vi "scan.vi"() -> (1 "载具码":string)   [LabVIEW 2014]
panel:
  in  "退出":bool
  in  "扫码控制键":bool
  in  "识别载具信息":string
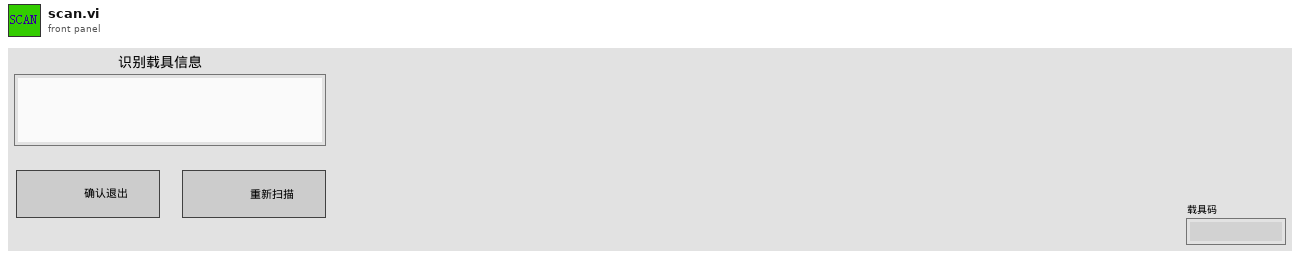
[diagram p1: front panel]
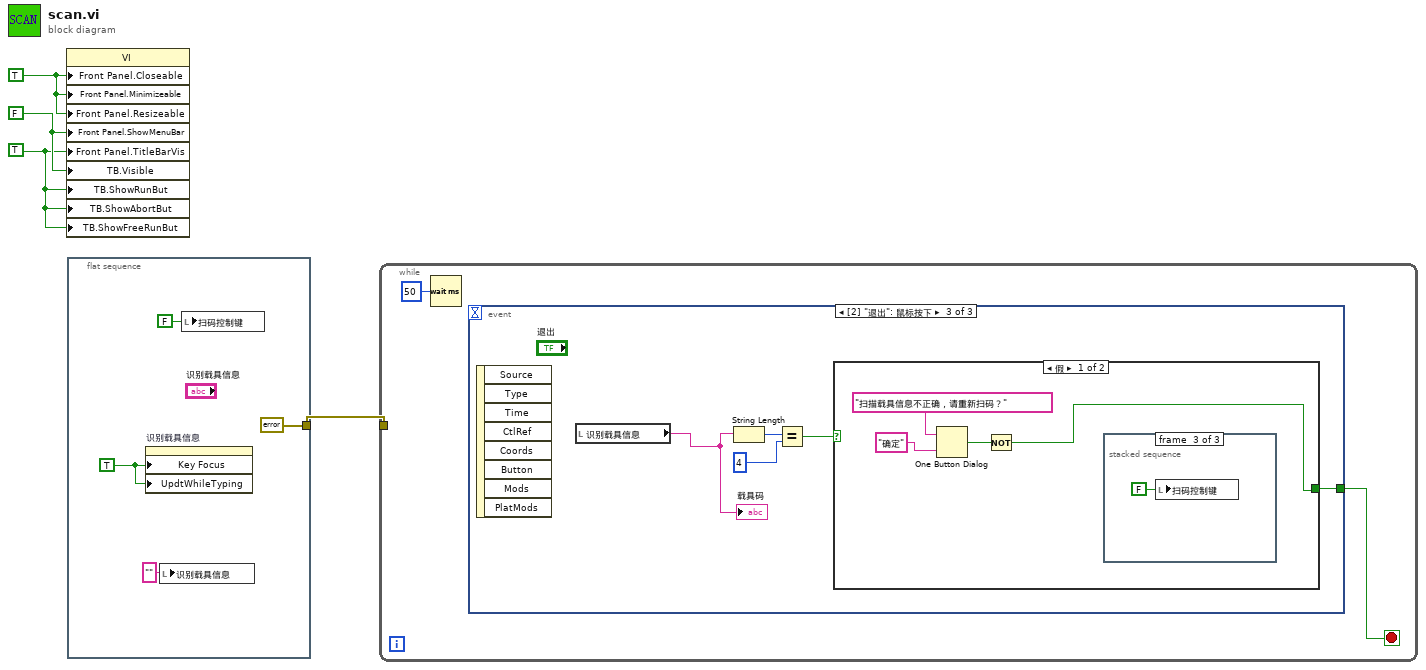
[diagram p0: block diagram]
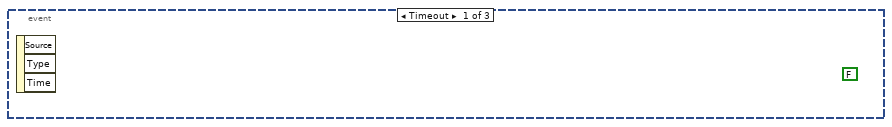
[diagram p2: hidden frame]
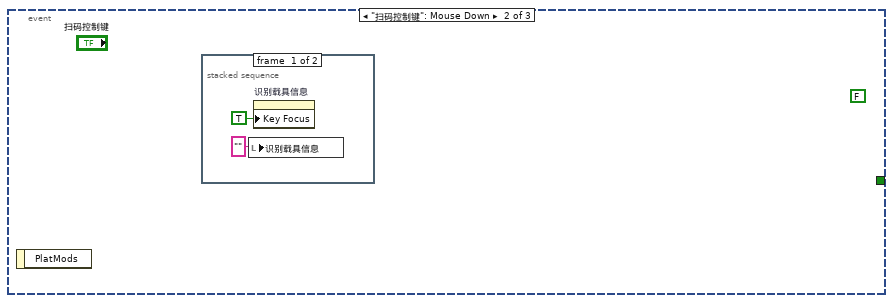
[diagram p3: hidden frame]
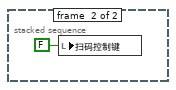
[diagram p4: hidden frame]
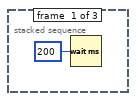
[diagram p5: hidden frame]
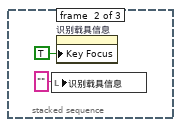
[diagram p6: hidden frame]
diagram:
  w2 = TRUE ("前面板窗口:可关闭")
  w1 = TRUE ("前面板窗口:可关闭")
  w3 = FALSE ("Front Panel Window:Closeable")
  n1 = property class="VI"("Front Panel.Closeable"=w1, "Front Panel.Minimizeable"=w1, "Front Panel.Resizeable"=w1, "Front Panel.ShowMenuBar"=w3, "Front Panel.TitleBarVis"=w2, "TB.Visible"=w3, "TB.ShowRunBut"=w2, "TB.ShowAbortBut"=w2, "TB.ShowFreeRunBut"=w2) -> ()  [unwired: 2 in, 2 out]
  n2 = flat-sequence {
    tunnel: [errorcluster {"status"=FALSE, "code"=0, "source"=""} ("错误常量")] -> w4
    frame #0 {
      w5 = TRUE ("键选中")
      n3 = property on="识别载具信息" class="Str"("Key Focus"=w5, "UpdtWhileTyping"=w5) -> ()  [unwired: 2 in, 2 out]
      n4 = local write "识别载具信息"("" ("扫码信息")) -> ()
      n5 = local write "扫码控制键"(FALSE ("扫码控制键")) -> ()
    }
  }
  n6 = while {
    tunnel: w4 -> [_]
    stop <- w9 stop-if-true
    n7 = Wait (ms)(milliseconds to wait=u32 50 ("等待时间（毫秒）")) -> ()  [unwired: 1 out]
    n8 = event shown="[2] \"退出\": 鼠标按下" {
      selector: _ -> [_ _ _]
      dyn-events: _ -> [_ _ _]
      timeout: _ -> [_ _ _]
      tunnel: [_ _ w18] -> w9
      event Timeout {
        (unwired) FALSE
        n9 = event-data() -> ()  [unwired: 1 in, 3 out]
      }
      event "扫码控制键": Mouse Down {
        (unwired) FALSE
        n10 = event-data() -> ()  [unwired: 1 in, 1 out]
        n11 = stacked-sequence {
          frame #0 {
            n12 = local write "识别载具信息"("" ("扫码信息")) -> ()
            n13 = property on="识别载具信息" class="Str"("Key Focus"=TRUE ("键选中")) -> ()  [unwired: 2 in, 2 out]
          }
          frame #1 {
            n14 = local write "扫码控制键"(FALSE ("扫码控制键")) -> ()
          }
        }
      }
      event "退出": Mouse Down {
        n15 = event-data() -> ()  [unwired: 1 in, 8 out]
        n16 = local read "识别载具信息"() -> (w14:string)
        "载具码" <- w14
        n17 = String Length(string=w14) -> (length=w16:i32)
        n18 = Equal?(x=w16, y=4) -> (x = y?=w17:bool)
        n19 = case shown="假" w17 {
          selector: w17 -> [_ w27]
          tunnel: [w22 w27] -> w18
          frame False {
            n20 = One Button Dialog(message="扫描载具信息不正确，请重新扫码？" ("消息"), button name ("OK")="确定" ("T按钮名称（“确定”）")) -> (true=w19:bool)
            n21 = Not(x=w19) -> (.not. x?=w22:bool)
            n22 = stacked-sequence {
              frame #0 {
                n23 = Wait (ms)(milliseconds to wait=u32 200 ("等待时间（毫秒）")) -> ()  [unwired: 1 out]
              }
              frame #1 {
                n24 = local write "识别载具信息"("" ("扫码信息")) -> ()
                n25 = property on="识别载具信息" class="Str"("Key Focus"=TRUE ("键选中")) -> ()  [unwired: 2 in, 2 out]
              }
              frame #2 {
                n26 = local write "扫码控制键"(FALSE ("扫码控制键")) -> ()
              }
            }
          }
          frame True {
          }
        }
      }
    }
  }
